vi "onNewHttpSession.vi"(6 "verify server (true)":bool, 7 "cookie file":path, 8 "error in (no error)":errorcluster, 9 "password":string, 10 "username":string, 11 "basic-http-client in":refnum<class "HttpClient.Basic.lvclass">) -> (0 "error out":errorcluster, 3 "basic-http-client out":refnum<class "HttpClient.Basic.lvclass">)   [LabVIEW 2020, in "httpClient.lvlib" / "HttpClient.Basic.lvclass"]
uses:
  HttpClient.Basic.lvclass
  HttpClient.Basic.lvclass/HttpClient.Basic.ctl
  <vilib>/httpClient/LabVIEWHTTPClient.lvlib
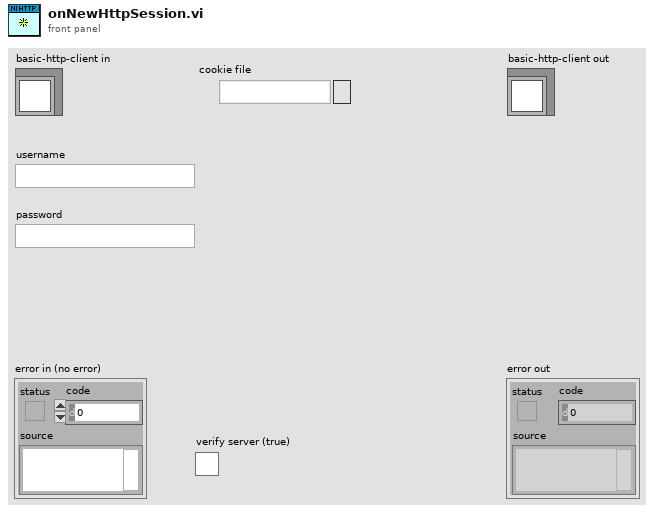
[diagram p1: front panel]
types:
  T1 = typedef "LabVIEWHTTPClient.lvlib/ClientHandle.ctl" = refnum<k1>
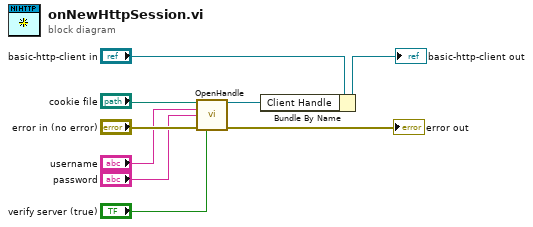
[diagram p0: block diagram]
diagram:
  n1 = call <vilib>:"OpenHandle.vi"("cookie file"="cookie file", "username"="username", "password"="password", "error in (no error)"="error in (no error)", "verify server(true)"="verify server (true)") -> ("client handle out"=w8:T1, "error out"=→"error out":errorcluster)  [unwired: 9 in]
  n2 = Bundle By Name(cluster="basic-http-client in", "Client Handle"=w8) -> (→"basic-http-client out":refnum<class "HttpClient.Basic.lvclass">)
